vi "MinValue.vi"(0 "CurrentMin":dbl, 3 "NewValue":dbl) -> (8 "Min":dbl)   [LabVIEW 2016]
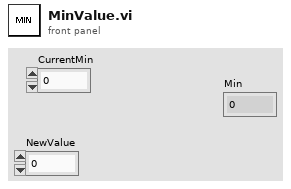
[diagram p1: front panel]
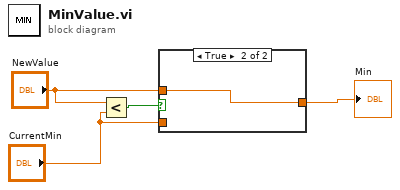
[diagram p0: block diagram]
diagram:
  n1 = Less?(x="NewValue", y="CurrentMin") -> (x < y?=w4:bool)
  n2 = case shown="True" w4 {
    tunnel: "NewValue" -> [_ w6]
    tunnel: [w5 w6] -> w2
    tunnel: "CurrentMin" -> [w5 _]
    frame False {
    }
    frame True {
    }
  }
  "Min" <- w2
